vi "Prepare State Logic.vi"(8 "error in (no error)":errorcluster, 11 "CIFCorePlugin in":refnum<class "CIFCorePlugin.lvclass">) -> (0 "error out":errorcluster, 2 "Prepare State Logic":T1, 3 "CIFCorePlugin out":refnum<class "CIFCorePlugin.lvclass">)   [LabVIEW 2021, in "CIFCorePlugin.lvclass"]
uses:
  CIFCorePlugin.lvclass
  CIFCorePlugin.lvclass/CIFCorePlugin.ctl
  Typedef/Prepare State Logic.ctl
  Common/Typedef/Plugin State.ctl
  Common/CIFCoreCommon.lvlib
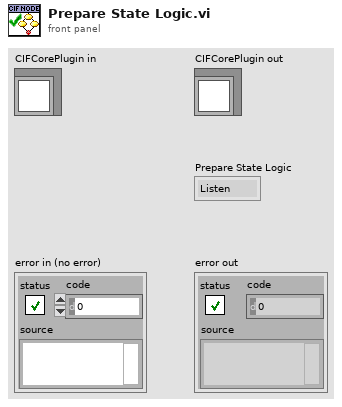
[diagram p1: front panel]
types:
  T1 = typedef "CIFCorePlugin.lvclass/Prepare State Logic.ctl" = enum16{"Listen", "Prepare", "Error", "Destroy"}
  T2 = typedef "CIFCorePlugin.lvclass/Energized States.ctl" = enum16{"Listen", "Prepare", "Execute", "Housekeep", "Cleanup", "Destroy"}
  T3 = typedef "CIFCoreCommon.lvlib/Plugin State.ctl" = enum32{"Null", "Creating", "Listening", "Running", "CleaningUp", "Destroying"}
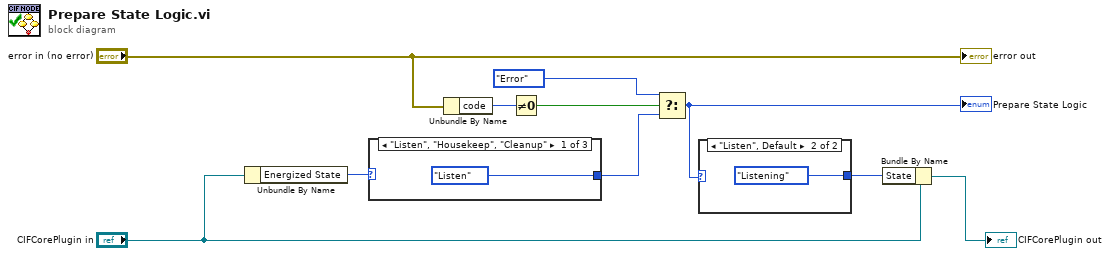
[diagram p0: block diagram]
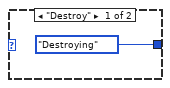
[diagram p2: hidden frame]
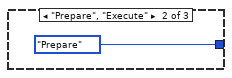
[diagram p3: hidden frame]
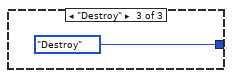
[diagram p4: hidden frame]
diagram:
  n1 = Unbundle By Name("CIFCorePlugin in") -> ("Energized State"=w6:T2)
  n2 = case shown="\"Listen\", \"Housekeep\", \"Cleanup\"" w6 {
    tunnel: [Prepare_State_Logic."Listen" ("Prepare State Logic") Prepare_State_Logic."Prepare" ("Prepare State Logic") Prepare_State_Logic."Destroy" ("Prepare State Logic")] -> w5
    frame "Listen", "Housekeep", "Cleanup" {
    }
    frame "Prepare", "Execute" {
    }
    frame "Destroy" {
    }
  }
  n3 = Unbundle By Name("error in (no error)") -> ("code"=w9:i32)
  n4 = Not Equal To 0?(x=w9) -> (x != 0?=w8:bool)
  n5 = Select(t=Prepare_State_Logic."Error" ("Prepare State Logic"), s=w8, f=w5) -> (s? t:f=w4:T1)
  "Prepare State Logic" <- w4
  n6 = case shown="\"Listen\", Default" w4 {
    tunnel: [Plugin_State."Destroying" ("Status.State") Plugin_State."Listening" ("Status.State")] -> w1
    frame "Destroy" {
    }
    frame "Listen", Default {
    }
  }
  n7 = Bundle By Name(cluster="CIFCorePlugin in", "State"=w1) -> (→"CIFCorePlugin out":refnum<class "CIFCorePlugin.lvclass">)
  "error out" <- "error in (no error)"
